vi "Wait Until Digital Comparison.vi"(0 "Device ID":T3(ring), 2 "Wait Until":enum8{"Is High", "Is Low"}(ring), 5 "Module":T1(ring), 7 "Digital_Input":T2(ring), 11 "error in":errorcluster, 13 "Time Out (10)":dbl=10.0) -> (4 "Device ID Out":T3(ring), 15 "error out":errorcluster)   [LabVIEW 2010]
doc: "This VI waits until a user-defined digital comparison is read."
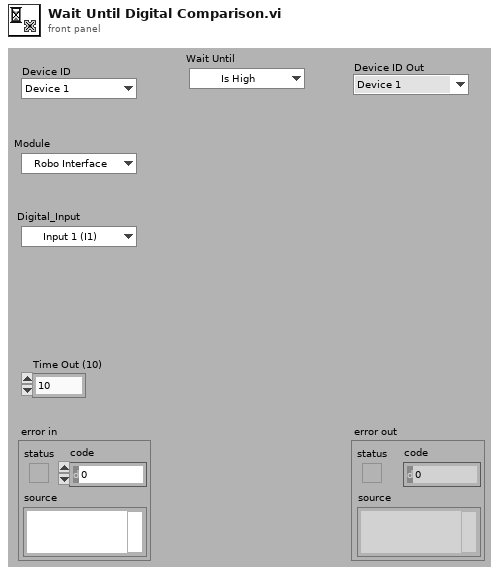
[diagram p1: front panel]
types:
  T1 = enum8{"Robo Interface", "Extension 1", "Extension 2", "Extension 3"}
  T2 = enum8{"Input 1 (I1)", "Input 2 (I2)", "Input 3 (I3)", "Input 4 (I4)", "Input 5 (I5)", "Input 6 (I6)", "Input 7 (I7)", "Input 8 (I8)"}
  T3 = enum16{"Device 1", "Device 2", "Device 3", "Device 4", "Device 5", "Device 6", "Device 7", "Device 8"}
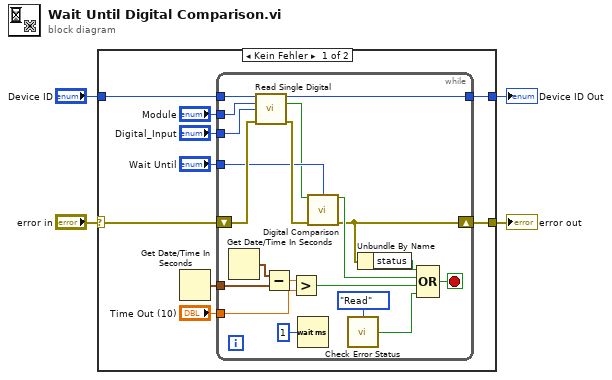
[diagram p0: block diagram]
diagram:
  n1 = case shown="Kein Fehler" "error in" {
    selector: "error in" -> [w6 w35]
    tunnel: [w5 w35] -> w3
    tunnel: "Device ID" -> [w8 w34]
    tunnel: [w7 w34] -> w1
    frame No Error {
      n2 = Get Date/Time In Seconds() -> (seconds since 1Jan1904=w12:timestamp)
      n3 = while {
        tunnel: "Wait Until" -> [w17]
        tunnel: w12 -> [w32]
        tunnel: "Time Out (10)" -> [w30]
        tunnel: w8 -> [w26]
        tunnel: "Module" -> [w25]
        tunnel: "Digital_Input" -> [w24]
        tunnel: [w23] -> w7
        shift-right: [w18] -> w5
        shift-left: w6 -> [w22]
        stop <- w28 stop-if-true
        n4 = Get Date/Time In Seconds() -> (seconds since 1Jan1904=w33:timestamp)
        n5 = call "Read Single Digital.vi"("Device ID"=w26, "Module"=w25, "Digital_Input"=w24, "error in"=w22) -> ("Device ID Out"=w23:T3, "Value"=w16:bool, "error out"=w19:errorcluster)  [unwired: 9 out]
        n6 = Subtract(x=w33, y=w32) -> (x-y=w31:dbl)
        n7 = Greater?(x=w31, y=w30) -> (0:w29:bool)
        n8 = Wait (ms)(milliseconds to wait=u32 1) -> ()  [unwired: 1 out]
        n9 = call "Digital Comparison.vi"("Data"=w16, "Wait Until"=w17, "error in"=w19) -> ("Result"=w20:bool, "error out"=w18:errorcluster)  [unwired: 11 out]
        n10 = call "Check Error Status.vi"("Action (Write)"=enum16{"Write", "Read"}."Read") -> ("Error?"=w14:bool)  [unwired: 2 in, 12 out]
        n11 = Unbundle By Name(w18) -> ("status"=w21:bool)
        n12 = Compound Arithmetic op=OR(w21, w20, w29, w14) -> (w28:bool)
      }
    }
    frame Error {
    }
  }
  "error out" <- w3
  "Device ID Out" <- w1
